vi "SampleGetIDMultiple.vi"() -> ()   [LabVIEW 2009]
panel:
  out "Identification List":string[](array[string])
  out "DeviceKey List Out":string[](array[string])
  out "error out":errorcluster
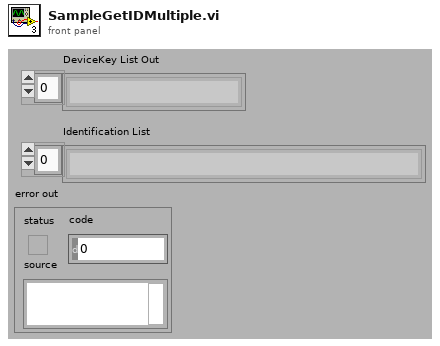
[diagram p1: front panel]
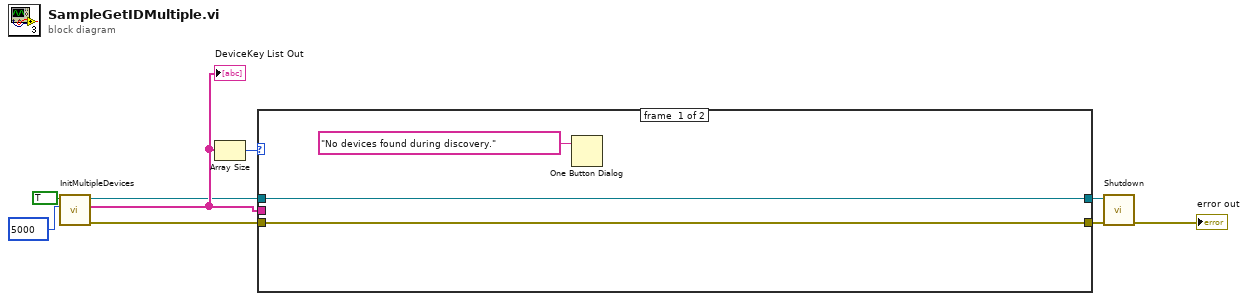
[diagram p0: block diagram]
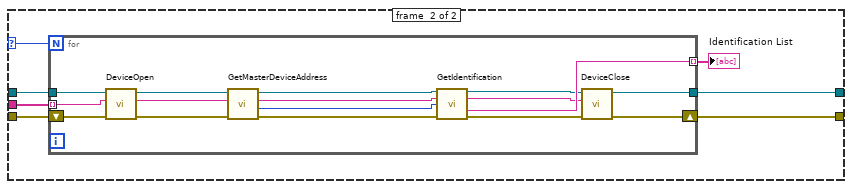
[diagram p2: hidden frame]
diagram:
  n1 = call "InitMultipleDevices.vi"("msecDelayForDiscovery"=5000, "logging"=TRUE) -> ("error out"=w3:errorcluster, "DeviceKey List Out"=w5:string[], "CmdLib Out"=w4:refnum<k24>)  [unwired: 3 in]
  "DeviceKey List Out" <- w5
  n2 = Array Size(array=w5) -> (size(s)=w6:i32)
  n3 = case shown="1, Default" w6 {
    selector: w6 -> [_ w19]
    tunnel: w5 -> [_ w18]
    tunnel: w4 -> [w11 w17]
    tunnel: w3 -> [w12 w16]
    tunnel: [w12 w15] -> w2
    tunnel: [w11 w14] -> w1
    frame #0 {
      n4 = One Button Dialog(message="No devices found during discovery.") -> ()  [unwired: 1 in, 1 out]
    }
    frame #1 {
      n5 = for {
        N: w19 -> [_]
        tunnel: w18 -> [w31] mode=indexing
        tunnel: [w35] -> w13 mode=indexing
        tunnel: w17 -> [w34]
        tunnel: [w33] -> w14
        shift-right: [w29] -> w15
        shift-left: w16 -> [w30]
        n6 = call "DeviceOpen.vi"("error in (no error)"=w30, "DeviceKey In"=w31, "CmdLib In"=w34) -> ("error out"=w24:errorcluster, "DeviceKey Out"=w25:string, "CmdLib Out"=w26:refnum<k24>)  [unwired: 2 in]
        n7 = call "GetMasterDeviceAddress.vi"("error in (no error)"=w24, "DeviceKey In"=w25, "CmdLib In"=w26) -> ("error out"=w20:errorcluster, "Device Address"=w23:i32, "DeviceKey Out"=w22:string, "CmdLib Out"=w21:refnum<k24>)  [unwired: 1 in]
        n8 = call "GetIdentification.vi"("CmdLib In"=w21, "DeviceKey In"=w22, "Device Address In"=w23, "error in (no error)"=w20) -> ("CmdLib Out"=w32:refnum<k24>, "DeviceKey Out"=w27:string, "Identification"=w35:string, "error out"=w28:errorcluster)  [unwired: 7 in, 1 out]
        n9 = call "DeviceClose.vi"("error in (no error)"=w28, "DeviceKey In"=w27, "CmdLib In"=w32) -> ("error out"=w29:errorcluster, "CmdLib Out"=w33:refnum<k24>)  [unwired: 2 in, 1 out]
      }
      "Identification List" <- w13
    }
  }
  n10 = call "Shutdown.vi"("error in (no error)"=w2, "CmdLib In"=w1) -> ("error out"=→"error out":errorcluster)  [unwired: 4 in, 1 out]
